vi "MSScript_SubVI_GetArrayIndexValue.vi"(10 "Index":i32[](array[numeric]), 11 "@name":string) -> (0 "Value Error?":bool, 1 "ArrayVariable out":ext[](array[numeric]), 2 "Is a variable ?":bool)   [LabVIEW 2018, in "MSScript.lvclass"]
uses:
  MSScript/MSScript.lvclass
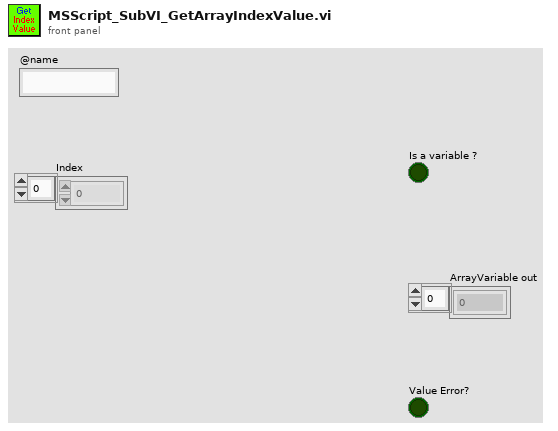
[diagram p1: front panel]
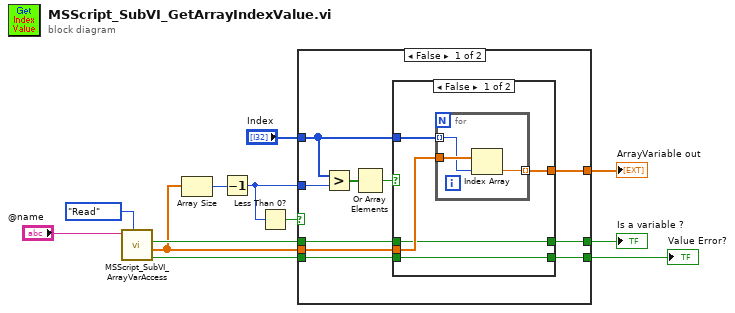
[diagram p0: block diagram]
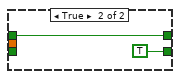
[diagram p2: hidden frame]
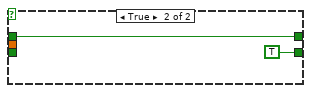
[diagram p3: hidden frame]
diagram:
  n1 = call "MSScript_SubVI_ArrayVarAccess.vi"("Function (Read)"=enum16{"Init", "Write", "Read"}."Read", "VarName"="@name") -> ("Value Error?"=w6:bool, "ArrayVariable out"=w5:ext[], "Is a variable ?"=w7:bool)  [unwired: 5 in]
  n2 = Array Size(array=w5) -> (size(s)=w10:i32)
  n3 = Decrement(x=w10) -> (x-1=w8:i32)
  n4 = Less Than 0?(x=w8) -> (x < 0?=w9:bool)
  n5 = case shown="False" w9 {
    tunnel: "Index" -> [w20 _]
    tunnel: [w22 _] -> w1
    tunnel: w5 -> [w21 _]
    tunnel: w7 -> [w17 w34]
    tunnel: [w16 w34] -> w3
    tunnel: w6 -> [w15 _]
    tunnel: [w14 TRUE ("Value Error?")] -> w2
    tunnel: w8 -> [w19 _]
    frame False {
      n6 = Greater?(x=w20, y=w19) -> (0:w18:bool[])
      n7 = Or Array Elements(Boolean array=w18) -> (logical OR=w13:bool)
      n8 = case shown="False" w13 {
        tunnel: [w27 _] -> w22
        tunnel: w21 -> [w26 _]
        tunnel: w20 -> [w23 _]
        tunnel: w17 -> [w25 w32]
        tunnel: [w25 w32] -> w16
        tunnel: w15 -> [w24 _]
        tunnel: [w24 TRUE ("Value Error?")] -> w14
        frame False {
          n9 = for {
            tunnel: w23 -> [w29] mode=indexing
            tunnel: w26 -> [w30]
            tunnel: [w28] -> w27 mode=indexing
            n10 = Index Array(array=w30, index=w29) -> (element=w28:ext)
          }
        }
        frame True {
        }
      }
    }
    frame True {
    }
  }
  "Is a variable ?" <- w3
  "Value Error?" <- w2
  "ArrayVariable out" <- w1
